vi "RGB Camera.vi"(8 "error in":errorcluster, 10 "RGB Camera Session":refnum<k21> caption="IMAQdx Session", 11 "Data":T1={"HTTP Queue"=refnum, "Notifier"=refnum, "Photo Save Directory"=path "", "Photo Period (ms)"=0, "Cameras Enabled"={"rgb_camera"=TRUE, "hsi_camera"=TRUE}, "Config ID"=0, "Server Address"=""}) -> (0 "error out":errorcluster)   [LabVIEW 2025]
doc: "Main VI for RGB camera. Inventory ID: 50065895s"
uses:
  defs/Data.ctl
  defs/HTTP Queue Definition.ctl
  defs/Notification Definition.ctl
  <vilib>/vision/driver/NI_Vision_Acquisition_Software.lvlib
panel:
  in  "Stop":bool
  out "RGB Image":T2(plugin-control)
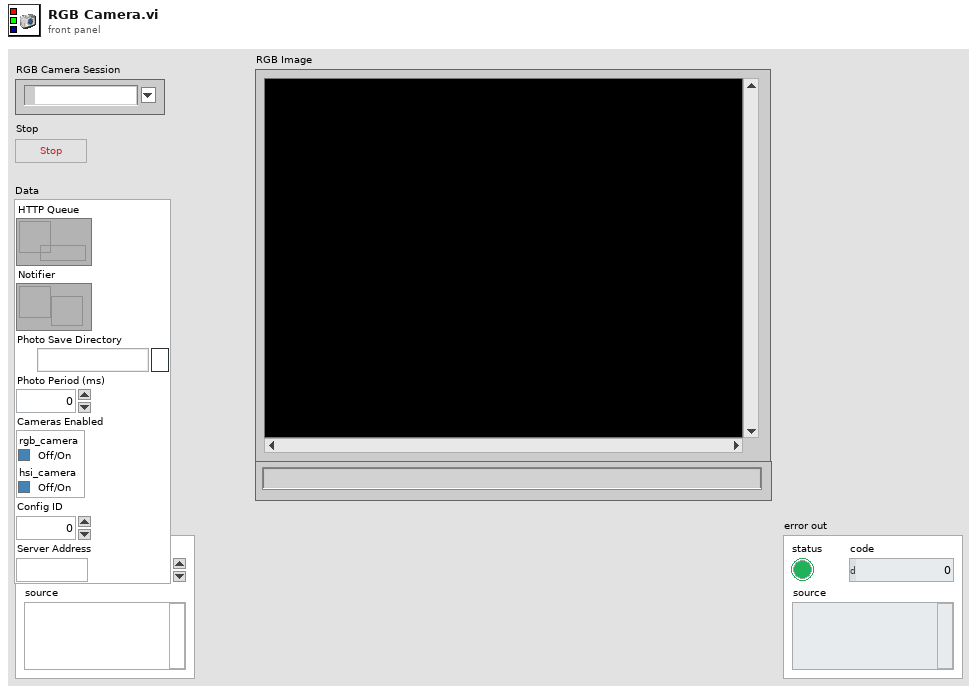
[diagram p1: front panel]
types:
  T1 = typedef "Data.ctl" = cluster{"HTTP Queue":refnum<queue>, "Notifier":refnum<notifier>, "Photo Save Directory":path, "Photo Period (ms)":u32, "Cameras Enabled":cluster{"rgb_camera":bool, "hsi_camera":bool}, "Config ID":u32, "Server Address":string}
  T2 = typedef "IMAQ Image.ctl" = refnum<image>
  T3 = typedef "Image Type" = u32
  T4 = typedef "IMAQdx.ctl" = refnum<k21>
  T5 = typedef "HTTP Queue Definition.ctl" = cluster{"Message":string, "Photo Path":path}
  T6 = typedef "Notification Definition.ctl" = cluster{"Message":string}
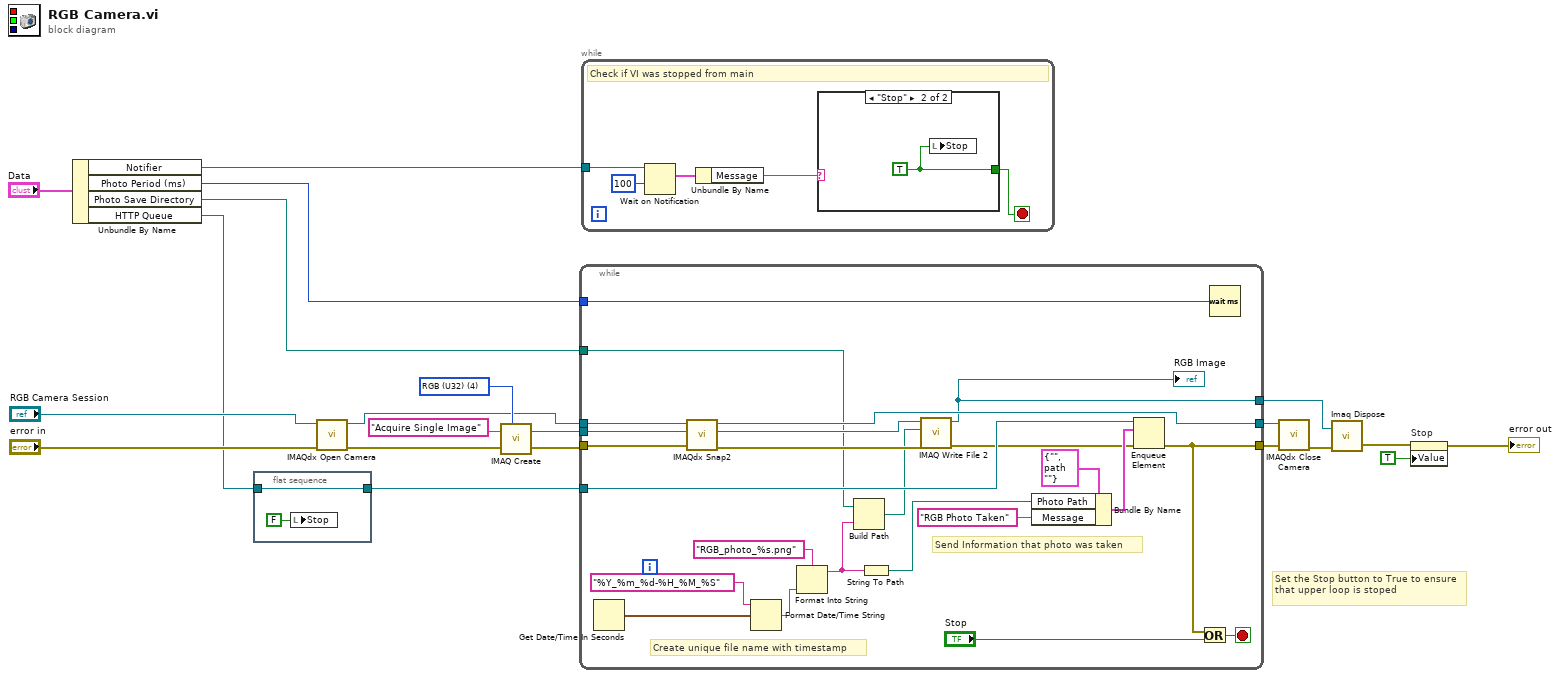
[diagram p0: block diagram]
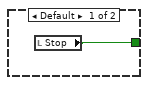
[diagram p2: hidden frame]
diagram:
  w16 = T3 4 items=["Grayscale (U8)", "Grayscale (I16)", "Grayscale (SGL)", "Complex (CSG)", "RGB (U32)", "HSL (U32)", "RGB (U64)", "Grayscale (U16)"] ("Image Type")
  # "Set the Stop button to True to ensure that upper loop is stoped"
  n1 = Unbundle By Name("Data") -> ("Notifier"=w4:refnum<notifier>, "Photo Period (ms)"=w3:u32, "Photo Save Directory"=w2:path, "HTTP Queue"=w1:refnum<queue>)
  n2 = flat-sequence {
    tunnel: w1 -> [w22]
    tunnel: [w22] -> w6
    frame #0 {
      n3 = local write "Stop"(FALSE ("Stop")) -> ()
    }
  }
  n4 = call <vilib>:"IMAQdx Open Camera.vi"("error in"="error in", "Session In"="RGB Camera Session") -> ("error out"=w15:errorcluster, "Session Out"=w11:T4)  [unwired: 1 in, 7 out]
  n5 = call "IMAQ Create"("Image Name"="Acquire Single Image", "Image Type"=w16, "error in (no error)"=w15) -> ("New Image"=w18:T2, "error out"=w14:errorcluster)  [unwired: 1 in, 1 out]
  n6 = while {
    tunnel: w14 -> [w44]
    tunnel: [w27] -> w13
    tunnel: w11 -> [w46]
    tunnel: [w42] -> w20
    tunnel: w18 -> [w45]
    tunnel: [w34] -> w21
    tunnel: w3 -> [w39]
    tunnel: w2 -> [w26]
    tunnel: w6 -> [w33]
    stop <- w41 stop-if-true
    # "Send Information that photo was taken"
    # "Create unique file name with timestamp"
    n7 = Get Date/Time In Seconds() -> (seconds since 1Jan1904=w37:timestamp)
    n8 = call <vilib>:"IMAQdx Snap2.vi"("error in"=w44, "Image In"=w45, "Session In"=w46) -> ("error out"=w43:errorcluster, "Image Out"=w47:T2, "Session Out"=w42:T4)  [unwired: 6 in]
    n9 = Format Date/Time String(time format string (%c)="%Y_%m_%d-%H_%M_%S", seconds (now)=w37) -> (date/time string=w35:string)  [unwired: 1 in]
    n10 = Format Into String(format string="RGB_photo_%s.png", w35) -> (resulting string=w25:string)  [unwired: 2 in, 1 out]
    n11 = Build Path(base path=w26, name or relative path=w25) -> (appended path=w30:path)
    n12 = String To Path(string=w25) -> (path=w24:path)
    n13 = call-poly "IMAQ Write File 2"("error in (no error)"=w43, "File Path"=w30, "Image"=w47) -> ("error out"=w28:errorcluster, "Image Out (duplicate)"=w34:T2)  [unwired: 7 in]
    "RGB Image" <- w34
    n14 = Bundle By Name(cluster=T5 {"Message"="", "Photo Path"=path ""} ("element"), "Photo Path"=w24, "Message"="RGB Photo Taken") -> (w31:T5)
    n15 = Enqueue Element(queue=w33, element=w31, error in (no error)=w28) -> (error out=w27:errorcluster)  [unwired: 1 in, 2 out]
    n16 = Or(x=w27, y="Stop") -> (x .or. y?=w41:bool)
    n17 = Wait (ms)(milliseconds to wait=w39) -> ()  [unwired: 1 out]
  }
  n18 = while {
    tunnel: w4 -> [w52]
    stop <- w49 stop-if-true
    # "Check if VI was stopped from main"
    n19 = Wait on Notification(notifier=w52, timeout in ms (-1)=100) -> (notification=w51:T6)  [unwired: 2 in, 3 out]
    n20 = Unbundle By Name(w51) -> ("Message"=w50:string)
    n21 = case shown="\"Stop\"" w50 {
      tunnel: [w53 w54] -> w49
      frame Default {
        n22 = local read "Stop"() -> (w53:bool)
      }
      frame "Stop" {
        w54 = TRUE
        n23 = local write "Stop"(w54) -> ()
      }
    }
  }
  n24 = call <vilib>:"IMAQdx Close Camera.vi"("error in"=w13, "Session In"=w20) -> ("error out"=w12:errorcluster)  [unwired: 9 out]
  n25 = call "Imaq Dispose"("Image"=w21, "error in (no error)"=w12) -> ("error out"=w9:errorcluster)  [unwired: 4 in]
  n26 = property on="Stop" class="Bool (strict)"(error in=w9, "Value"=TRUE) -> (error out=→"error out":errorcluster)  [unwired: 1 in, 1 out]
